vi "CRYDelete All.vi"(7 "sAction":string="GetActiveSymbols", 10 "Type":enum16{"Curves", "Values", "Results", "WFM"}(ring), 11 "sNames":string[](array[string])) -> (1 "Delete?":bool=TRUE, 2 "Deleted Rows":i32[](array[numeric]))   [LabVIEW 2013]
panel:
  # "Delete  Data"
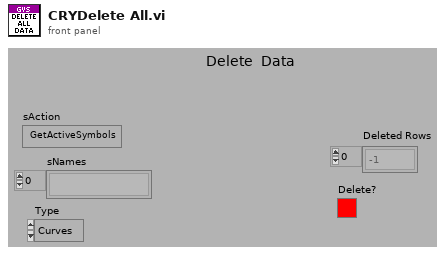
[diagram p1: front panel]
types:
  T1 = enum16{"Left Button", "Center Button", "Right Button", "Window Close"}
  T2 = enum16{"OK", "Yes", "YesNo", "YesNoCancel", "ReplaceAppend"}
  T3 = typedef "CRYData Cluster Array.ctl" = T4[]
  T4 = typedef "CRYData Cluster.ctl" = cluster{"Name":string, "Curve":cluster{"x":dbl, "y":dbl, "z":dbl}[], "X data":u16, "Y data":u16, "Z data":u16, "X axis":u16, "Y axis":u16, "Z axis":u16, "X unit":string, "Y unit":string, "Z unit":string, "X dB ref":dbl, "Y dB ref":dbl, "Z dB ref":dbl, "single val":bool, "protected":bool, "display X":bool, "display Y":bool, "display Z":bool, "Test Info":string, "Step No.":i32, "Plot Settings":cluster{"Color":u32, "Interpolation":u8, "Point Style":u8, "Line Style":u8, "Point Color":u32, "Line Width":u8, "Bar Plot Style":u8, "Fill To":i16}, "AutoProtect":bool}
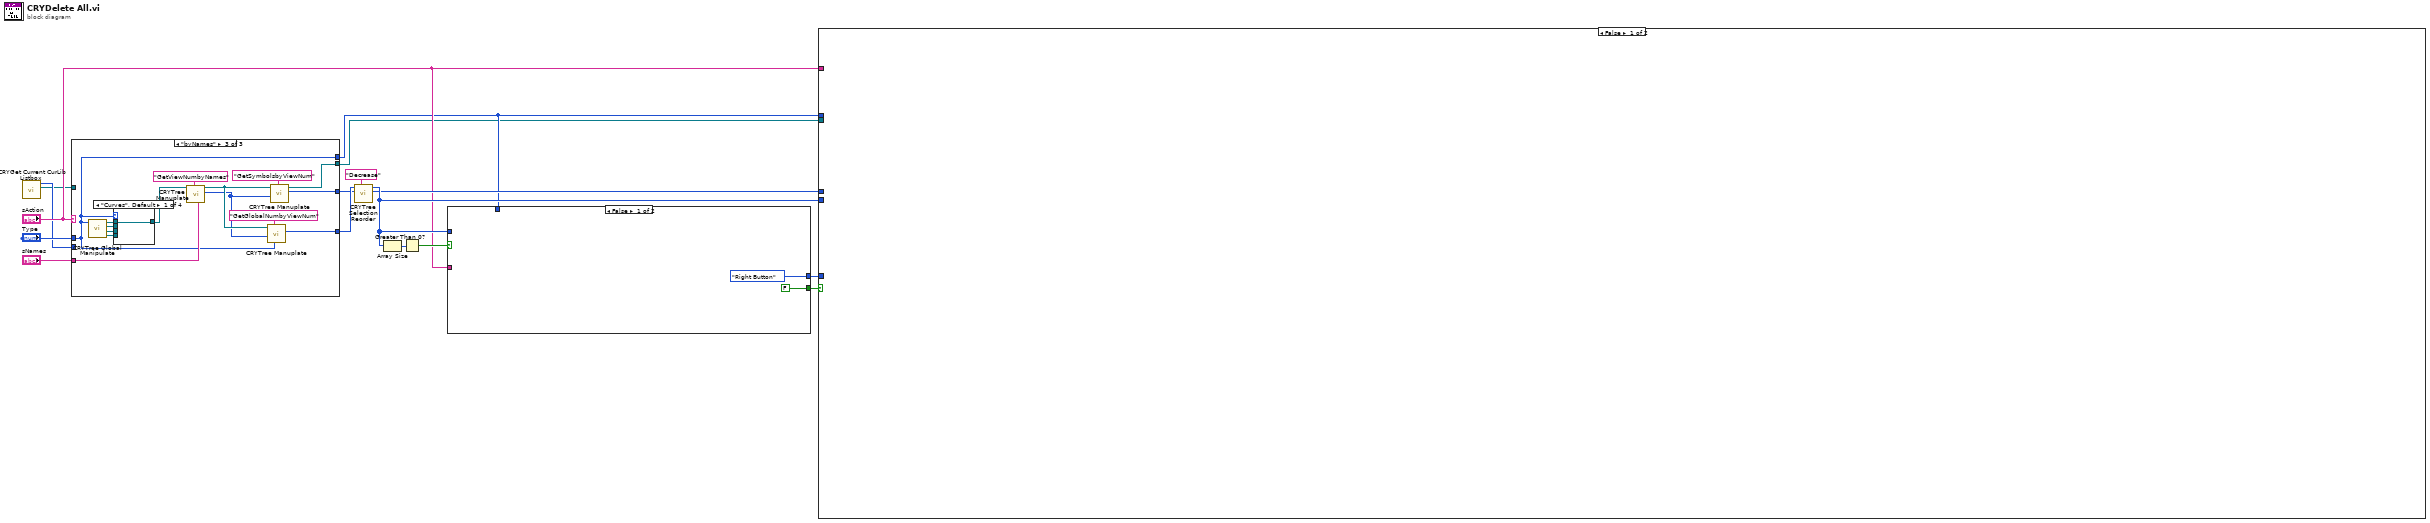
[diagram p0: block diagram]
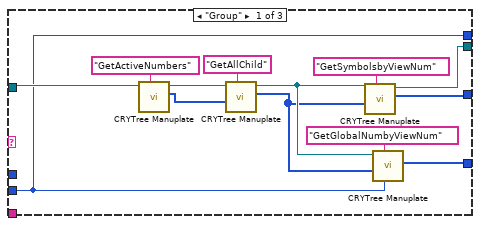
[diagram p2: hidden frame]
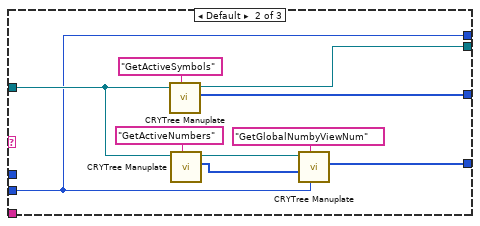
[diagram p3: hidden frame]
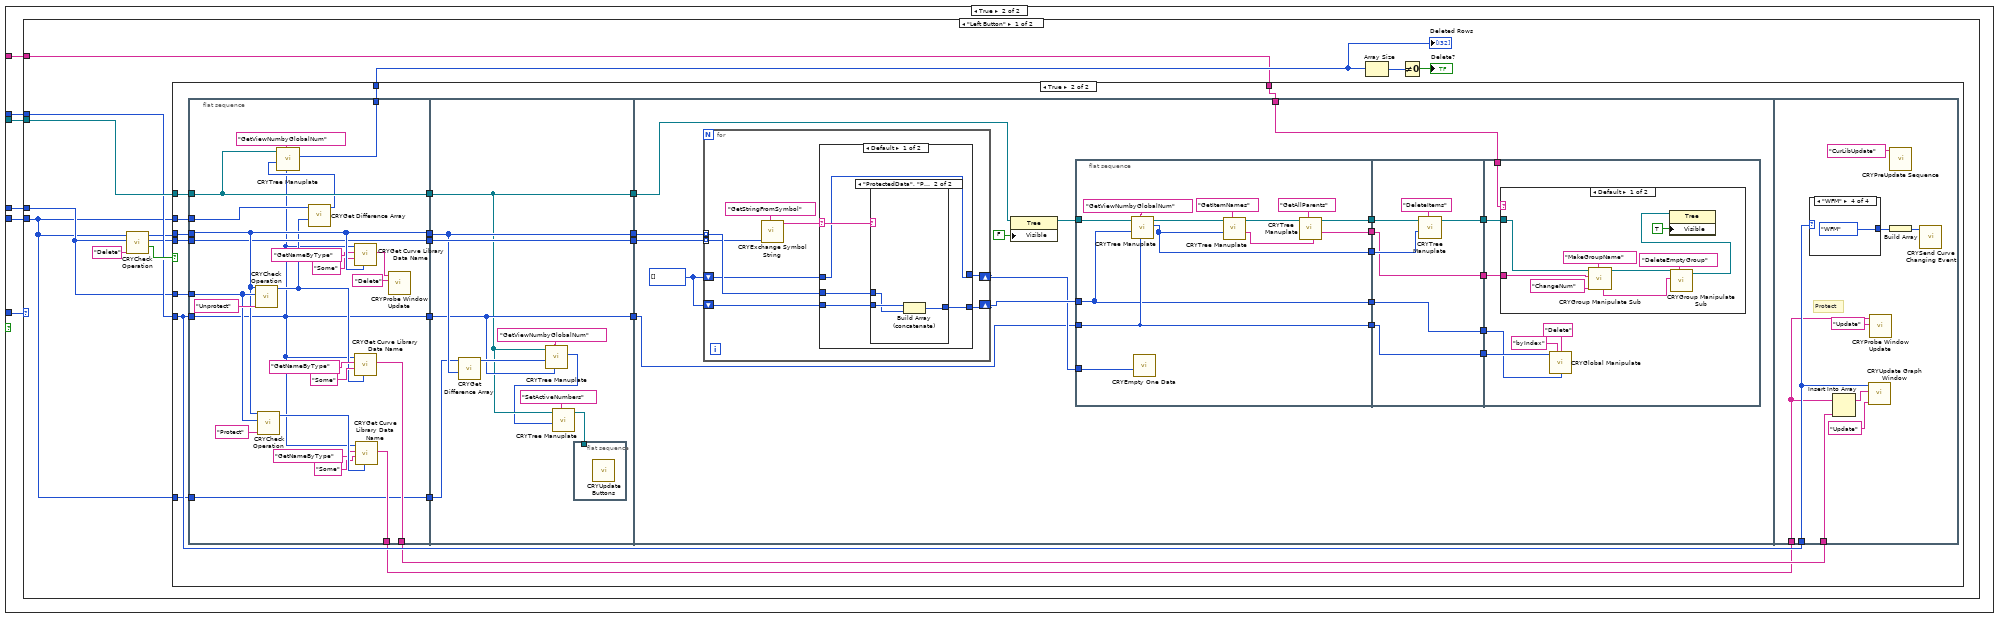
[diagram p7: hidden frame]
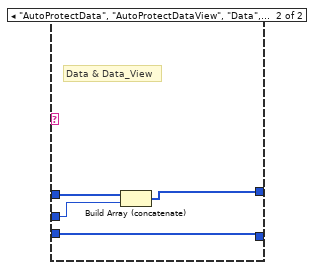
[diagram p11: hidden frame]
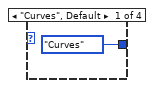
[diagram p12: hidden frame]
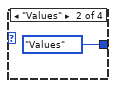
[diagram p13: hidden frame]
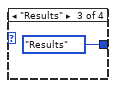
[diagram p14: hidden frame]
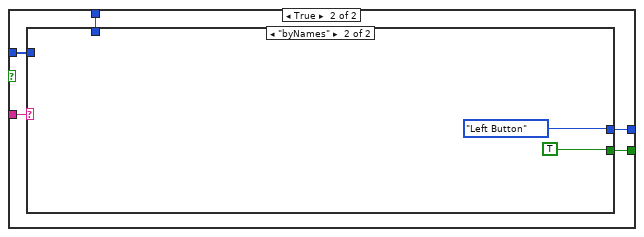
[diagram p16: hidden frame]
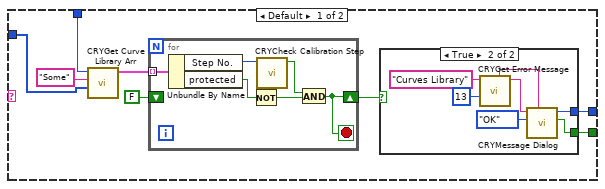
[diagram p17: hidden frame]
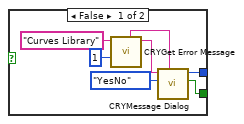
[diagram p18: hidden frame]
diagram:
  n1 = call "CRYGet Current CurLib Listbox.vi"() -> ("CurLib Tree"=w2:refnum<vi>, "Type"=w4:enum16{"Curves", "Values", "Results", "WFM"})  [unwired: 9 in, 1 out]
  n2 = case shown="\"byNames\"" "sAction" {
    tunnel: [w26 w37 w49] -> w10
    tunnel: w2 -> [w28 w36 _]
    tunnel: [w24 w32 w53] -> w12
    tunnel: w4 -> [w17 w30 _]
    tunnel: "sNames" -> [_ _ w47]
    tunnel: "Type" -> [_ _ w40]
    tunnel: [w18 w31 w41] -> w1
    tunnel: [w17 w30 w40] -> w3
    frame "Group" {
      n3 = call "CRYTree Manuplate.vi"("sAction"="GetActiveNumbers", "Tree in"=w28) -> ("nData Out"=w20:i32[], "Tree Out"=w22:refnum<vi>)  [unwired: 6 in, 2 out]
      n4 = call "CRYTree Manuplate.vi"("sAction"="GetAllChild", "nData"=w20, "Tree in"=w22) -> ("nData Out"=w19:i32[], "Tree Out"=w21:refnum<vi>)  [unwired: 5 in, 2 out]
      n5 = call "CRYTree Manuplate.vi"("sAction"="GetSymbolsbyViewNum", "nData"=w19, "Tree in"=w21) -> ("nData Out"=w26:i32[], "Tree Out"=w18:refnum<vi>)  [unwired: 5 in, 2 out]
      n6 = call "CRYTree Manuplate.vi"("Type"=w17, "sAction"="GetGlobalNumbyViewNum", "nData"=w19, "Tree in"=w21) -> ("nData Out"=w24:i32[])  [unwired: 4 in, 3 out]
    }
    frame Default {
      n7 = call "CRYTree Manuplate.vi"("sAction"="GetActiveSymbols", "Tree in"=w36) -> ("nData Out"=w37:i32[], "Tree Out"=w31:refnum<vi>)  [unwired: 6 in, 2 out]
      n8 = call "CRYTree Manuplate.vi"("sAction"="GetActiveNumbers", "Tree in"=w36) -> ("nData Out"=w33:i32[], "Tree Out"=w34:refnum<vi>)  [unwired: 6 in, 2 out]
      n9 = call "CRYTree Manuplate.vi"("Type"=w30, "sAction"="GetGlobalNumbyViewNum", "nData"=w33, "Tree in"=w34) -> ("nData Out"=w32:i32[])  [unwired: 4 in, 3 out]
    }
    frame "byNames" {
      n10 = call "CRYTree Global Manipulate.vi"("Type In"=w40) -> ("WFM Tree"=w43:refnum<vi>, "Results Tree"=w44:refnum<vi>, "Values Tree"=w45:refnum<vi>, "Tree/Curve Tree"=w46:refnum<vi>)  [unwired: 7 in]
      n11 = case shown="\"Curves\", Default" w40 {
        tunnel: w46 -> [w55 _ _ _]
        tunnel: [w55 w56 w57 w58] -> w42
        tunnel: w45 -> [_ w56 _ _]
        tunnel: w44 -> [_ _ w57 _]
        tunnel: w43 -> [_ _ _ w58]
        frame "Curves", Default {
        }
        frame "Values" {
        }
        frame "Results" {
        }
        frame "WFM" {
        }
      }
      n12 = call "CRYTree Manuplate.vi"("sData"=w47, "sAction"="GetViewNumbyNames", "Tree in"=w42) -> ("nData Out"=w48:i32[], "Tree Out"=w50:refnum<vi>)  [unwired: 5 in, 2 out]
      n13 = call "CRYTree Manuplate.vi"("Type"=w40, "sAction"="GetGlobalNumbyViewNum", "nData"=w48, "Tree in"=w50) -> ("nData Out"=w53:i32[])  [unwired: 4 in, 3 out]
      n14 = call "CRYTree Manuplate.vi"("sAction"="GetSymbolsbyViewNum", "nData"=w48, "Tree in"=w50) -> ("nData Out"=w49:i32[], "Tree Out"=w41:refnum<vi>)  [unwired: 5 in, 2 out]
    }
  }
  n15 = call "CRYTree Selection Reorder.vi"("sAction"="Decrease", "Symbol In"=w10, "Number In"=w12) -> ("Symbol Out"=w9:i32[], "Number Out"=w11:i32[])  [unwired: 7 in]
  n16 = Array Size(array=w11) -> (size(s)=w15:i32)
  n17 = Greater Than 0?(x=w15) -> (x > 0?=w14:bool)
  n18 = case shown="False" w14 {
    tunnel: [T1."Right Button" ("Which Button?") w65] -> w16
    tunnel: w11 -> [_ w64]
    tunnel: w3 -> [_ w63]
    tunnel: [FALSE ("YesNo") w62] -> w13
    tunnel: "sAction" -> [_ w61]
    frame False {
    }
    frame True {
      n19 = case shown="\"byNames\"" w61 {
        tunnel: [w73 T1."Left Button" ("Which Button?")] -> w65
        tunnel: w64 -> [w72 _]
        tunnel: w63 -> [w71 _]
        tunnel: [w66 TRUE ("YesNo")] -> w62
        frame Default {
          n20 = call "CRYGet Curve Library Arr.vi"("Index"=w72, "sOption"="Some", "Type In"=w71) -> ("Curves/Values"=w69:T3)  [unwired: 6 in, 2 out]
          n21 = for {
            tunnel: w69 -> [w93] mode=indexing
            shift-right: [w90] -> w67
            shift-left: FALSE -> [_]
            stop <- w90 stop-if-true
            n22 = Unbundle By Name(w93) -> ("Step No."=w92:i32, "protected"=w88:bool)
            n23 = Not(x=w88) -> (.not. x?=w89:bool)
            n24 = call "CRYCheck Calibration Step.vi"("Step No"=w92) -> ("Is Calibration?"=w91:bool)  [unwired: 9 in, 1 out]
            n25 = And(x=w91, y=w89) -> (x .and. y?=w90:bool)
          }
          n26 = case shown="True" w67 {
            tunnel: [w75 w82] -> w73
            tunnel: [w74 w81] -> w66
            frame False {
              n27 = call "CRYGet Error Message.vi"("Error No"=1, "Kind"="Curves Library") -> ("Message"=w77:string, "Window Title"=w76:string)  [unwired: 4 in, 4 out]
              n28 = call "CRYMessage Dialog.vi"("Window Title"=w76, "YesNoCancel"=T2."YesNo", "Message Content"=w77) -> ("YesNo"=w74:bool, "Which Button?"=w75:T1)  [unwired: 7 in]
            }
            frame True {
              n29 = call "CRYGet Error Message.vi"("Error No"=13, "Kind"="Curves Library") -> ("Message"=w84:string, "Window Title"=w83:string)  [unwired: 4 in, 4 out]
              n30 = call "CRYMessage Dialog.vi"("Window Title"=w83, "YesNoCancel"=T2."OK", "Message Content"=w84) -> ("YesNo"=w81:bool, "Which Button?"=w82:T1)  [unwired: 7 in]
            }
          }
        }
        frame "byNames" {
        }
      }
    }
  }
  n31 = case shown="False" w13 {
    tunnel: w16 -> [_ w101]
    tunnel: w9 -> [_ w100]
    tunnel: w1 -> [_ w99]
    tunnel: w11 -> [_ w98]
    tunnel: w3 -> [_ w97]
    tunnel: "sAction" -> [_ w96]
    frame False {
    }
    frame True {
      n32 = case shown="\"Left Button\"" w101 {
        tunnel: w100 -> [w107 _]
        tunnel: w98 -> [w103 _]
        tunnel: w99 -> [w110 _]
        tunnel: w97 -> [w109 _]
        tunnel: w96 -> [w102 _]
        frame "Left Button" {
          n33 = call "CRYCheck Operation.vi"("Operation"="Delete", "Item Symbols In"=w107, "Index Array In"=w103) -> ("Operation ?"=w113:bool, "Item Symbols Out"=w106:i32[], "Array Out"=w105:i32[])  [unwired: 1 in, 5 out]
          n34 = case shown="True" w113 {
            tunnel: w110 -> [_ w133]
            tunnel: w105 -> [_ w130]
            tunnel: w109 -> [_ w132]
            tunnel: w107 -> [_ w131]
            tunnel: w106 -> [_ w128]
            tunnel: w103 -> [_ w127]
            tunnel: w103 -> [_ w125]
            tunnel: [_ w124] -> w104
            tunnel: w102 -> [_ w114]
            frame False {
            }
            frame True {
              n35 = flat-sequence {
                tunnel: w132 -> [w135]
                tunnel: w130 -> [w149]
                tunnel: w133 -> [w137]
                tunnel: [w142] -> w123
                tunnel: [w137] -> w121
                tunnel: [w149] -> w119
                tunnel: [w135] -> w117
                tunnel: w131 -> [w151]
                tunnel: [w156] -> w126
                tunnel: [w157] -> w129
                tunnel: w128 -> [w142]
                tunnel: [w141] -> w115
                tunnel: w127 -> [w141]
                tunnel: w125 -> [w140]
                tunnel: [w134] -> w124
                tunnel: w123 -> [w167]
                tunnel: [w167] -> w122
                tunnel: w121 -> [w160]
                tunnel: [w160] -> w120
                tunnel: w119 -> [w166]
                tunnel: [w166] -> w118
                tunnel: w117 -> [w162]
                tunnel: [w162] -> w116
                tunnel: w115 -> [w165]
                tunnel: w122 -> [w185]
                tunnel: w120 -> [w179]
                tunnel: w118 -> [w186]
                tunnel: w116 -> [w181]
                tunnel: w114 -> [w177]
                tunnel: w126 -> [w248]
                tunnel: w132 -> [w252]
                tunnel: w129 -> [w250]
                frame #0 {
                  n36 = call "CRYCheck Operation.vi"("Operation"="Unprotect", "Item Symbols In"=w151, "Index Array In"=w149) -> ("Array Out"=w139:i32[])  [unwired: 6 in, 2 out]
                  n37 = call "CRYCheck Operation.vi"("Operation"="Protect", "Item Symbols In"=w151, "Index Array In"=w149) -> ("Array Out"=w150:i32[])  [unwired: 6 in, 2 out]
                  n38 = call "CRYGet Difference Array.vi"("Array 2"=w139, "Array 1"=w140) -> ("Diff Out"=w136:i32[])  [unwired: 3 in, 6 out]
                  n39 = call "CRYTree Manuplate.vi"("Type"=w135, "sAction"="GetViewNumbyGlobalNum", "nData"=w136, "Tree in"=w137) -> ("nData Out"=w134:i32[])  [unwired: 4 in, 3 out]
                  n40 = call "CRYGet Curve Library Data Name.vi"("nData"=w149, "sOption"="Some", "sAction"="GetNameByType", "Type"=w135) -> ("sNames"=w155:string[])  [unwired: 2 in, 5 out]
                  n41 = call "CRYGet Curve Library Data Name.vi"("nData"=w139, "sOption"="Some", "sAction"="GetNameByType", "Type"=w135) -> ("sNames"=w157:string[])  [unwired: 2 in, 5 out]
                  n42 = call "CRYGet Curve Library Data Name.vi"("nData"=w150, "sOption"="Some", "sAction"="GetNameByType", "Type"=w135) -> ("sNames"=w156:string[])  [unwired: 2 in, 5 out]
                  n43 = call "CRYProbe Window Update.vi"("sAction"="Delete", "Names"=w155) -> ()  [unwired: 2 in, 8 out]
                }
                frame #1 {
                  n44 = call "CRYGet Difference Array.vi"("Array 2"=w166, "Array 1"=w165) -> ("Diff Out"=w163:i32[])  [unwired: 3 in, 6 out]
                  n45 = call "CRYTree Manuplate.vi"("Type"=w162, "sAction"="GetViewNumbyGlobalNum", "nData"=w163, "Tree in"=w160) -> ("nData Out"=w159:i32[])  [unwired: 4 in, 3 out]
                  n46 = call "CRYTree Manuplate.vi"("sAction"="SetActiveNumbers", "nData"=w159, "Tree in"=w160) -> ("Tree Out"=w158:refnum<vi>)  [unwired: 5 in, 3 out]
                  n47 = flat-sequence {
                    tunnel: w158 -> [_]
                    frame #0 {
                      n48 = call "CRYUpdate Buttons.vi"() -> ()  [unwired: 1 in, 11 out]
                    }
                  }
                }
                frame #2 {
                  w184 = i32[] []
                  n49 = for {
                    tunnel: w186 -> [w230] mode=indexing
                    tunnel: w185 -> [w227] mode=indexing
                    shift-right: [w225] -> w182
                    shift-left: w184 -> [w226]
                    shift-right: [w223] -> w183
                    shift-left: w184 -> [w224]
                    n50 = call "CRYExchange Symbol String.vi"("nData"=w227, "sAction"="GetStringFromSymbol") -> ("sData out"=w228:string)  [unwired: 8 in, 1 out]
                    n51 = case shown="Default" w228 {
                      selector: w228 -> [w234 _]
                      tunnel: w230 -> [w235 w242]
                      tunnel: w226 -> [w231 w243]
                      tunnel: [w231 w241] -> w225
                      tunnel: w224 -> [w233 w240]
                      tunnel: [w232 w240] -> w223
                      frame Default {
                        n52 = case shown="\"ProtectedData\", \"ProtectedDataView\", \"ProtectedNoData\", \"ProtectedNoDataView\"" w234 {
                          tunnel: w235 -> [_ w237]
                          tunnel: w233 -> [w236 w239]
                          tunnel: [w236 w238] -> w232
                          frame Default {
                            # "NoData"
                            # "Nothing to do"
                          }
                          frame "ProtectedData", "ProtectedDataView", "ProtectedNoData", "ProtectedNoDataView" {
                            n53 = Build Array (concatenate)(w239, w237) -> (w238:i32[])
                          }
                        }
                      }
                      frame "AutoProtectData", "AutoProtectDataView", "Data", "DataView" {
                        # "Data & Data_View"
                        n54 = Build Array (concatenate)(w243, w242) -> (w241:i32[])
                      }
                    }
                  }
                  n55 = property class="Tree"(reference=w179, "Visible"=FALSE) -> (reference out=w178:refnum<vi>)  [unwired: 1 in, 1 out]
                  n56 = flat-sequence {
                    tunnel: w178 -> [w198]
                    tunnel: w183 -> [w196]
                    tunnel: w181 -> [w197]
                    tunnel: [w197] -> w176
                    tunnel: [w196] -> w174
                    tunnel: w182 -> [w195]
                    tunnel: [w189] -> w172
                    tunnel: [w192] -> w170
                    tunnel: [w187] -> w169
                    tunnel: w176 -> [w206]
                    tunnel: [w206] -> w175
                    tunnel: w174 -> [w205]
                    tunnel: [w205] -> w173
                    tunnel: w172 -> [w203]
                    tunnel: [w202] -> w171
                    tunnel: w170 -> [w201]
                    tunnel: w169 -> [w200]
                    tunnel: [w200] -> w168
                    tunnel: w175 -> [w211]
                    tunnel: w173 -> [w209]
                    tunnel: w171 -> [w208]
                    tunnel: w177 -> [w210]
                    tunnel: w168 -> [w207]
                    frame #0 {
                      n57 = call "CRYTree Manuplate.vi"("Type"=w197, "sAction"="GetViewNumbyGlobalNum", "nData"=w196, "Tree in"=w198) -> ("nData Out"=w192:i32[], "Tree Out"=w193:refnum<vi>)  [unwired: 4 in, 2 out]
                      n58 = call "CRYEmpty One Data.vi"("Index"=w195) -> ()  [unwired: 2 in, 9 out]
                      n59 = call "CRYTree Manuplate.vi"("sAction"="GetItemNames", "nData"=w192, "Tree in"=w193) -> ("sData Out"=w188:string[], "Tree Out"=w190:refnum<vi>)  [unwired: 5 in, 2 out]
                      n60 = call "CRYTree Manuplate.vi"("sData"=w188, "sAction"="GetAllParents", "Tree in"=w190) -> ("sData Out"=w187:string[], "Tree Out"=w189:refnum<vi>)  [unwired: 5 in, 2 out]
                    }
                    frame #1 {
                      n61 = call "CRYTree Manuplate.vi"("sAction"="DeleteItems", "nData"=w201, "Tree in"=w203) -> ("Tree Out"=w202:refnum<vi>)  [unwired: 5 in, 3 out]
                    }
                    frame #2 {
                      n62 = case shown="Default" w210 {
                        tunnel: w208 -> [w219 _]
                        tunnel: w207 -> [w216 _]
                        frame Default {
                          n63 = call "CRYGroup Manipulate Sub.vi"("sAction"="MakeGroupName", "sOption"="ChangeNum", "sData"=w216, "Tree in"=w219) -> ("Tree Out"=w217:refnum<vi>, "sData Out"=w214:string[])  [unwired: 3 in, 3 out]
                          n64 = call "CRYGroup Manipulate Sub.vi"("sAction"="DeleteEmptyGroup", "sData"=w214, "Tree in"=w217) -> ("Tree Out"=w215:refnum<vi>)  [unwired: 4 in, 4 out]
                          n65 = property class="Tree"(reference=w215, "Visible"=TRUE) -> ()  [unwired: 1 in, 2 out]
                        }
                        frame "Group" {
                        }
                      }
                      n66 = call "CRYGlobal Manipulate.vi"("Type"=w211, "sOption"="byIndex", "sAction"="Delete", "nData"=w209) -> ()  [unwired: 5 in, 7 out]
                    }
                  }
                }
                frame #3 {
                  # "Protect"
                  n67 = case shown="\"WFM\"" w252 {
                    tunnel: [enum16{"Curves", "Values", "Results", "WFM"}."Curves" ("Type In") enum16{"Curves", "Values", "Results", "WFM"}."Values" ("Type In") enum16{"Curves", "Values", "Results", "WFM"}."Results" ("Type In") enum16{"Curves", "Values", "Results", "WFM"}."WFM" ("Type In")] -> w246
                    frame "Curves", Default {
                    }
                    frame "Values" {
                    }
                    frame "Results" {
                    }
                    frame "WFM" {
                    }
                  }
                  n68 = Insert Into Array(array=w248, new element=w250) -> (w249:string[])  [unwired: 1 in]
                  n69 = call "CRYUpdate Graph Window.vi"("sOption"="Update", "Del/Update Names"=w249, "Type"=w252) -> ()  [unwired: 1 in, 8 out]
                  n70 = call "CRYProbe Window Update.vi"("sAction"="Update", "Names"=w248) -> ()  [unwired: 2 in, 8 out]
                  n71 = call "CRYPreUpdate Sequence.vi"("EventName"="CurLibUpdate") -> ()  [unwired: 15 in]
                  n72 = Build Array(w246) -> (w245:enum16{"Curves", "Values", "Results", "WFM"}[])
                  n73 = call "CRYSend Curve Changing Event.vi"("Type"=w245) -> ()  [unwired: 11 out]
                }
              }
            }
          }
          "Deleted Rows" <- w104
          n74 = Array Size(array=w104) -> (size(s)=w111:i32)
          n75 = Not Equal To 0?(x=w111) -> (x != 0?=→"Delete?":bool)
        }
        frame Default {
        }
      }
    }
  }
